vi "Check for Errors.vi"(8 "error in":errorcluster, 11 "Engine in":refnum<class "Engine.lvclass">) -> (0 "error out":errorcluster, 3 "Engine out":refnum<class "Engine.lvclass">)   [LabVIEW 2023, in "Engine.lvlib" / "Engine.lvclass"]
doc: "This routine checks incoming error terminals and relays an error event to the fault handler if there is an error, removing the error from the terminal and allowing the software to continue executing\n\n*This VI will allow the error to pass through if the original error event was not created."
uses:
  Project/Engine.lvclass
  C:/Users/Public/Documents/Development/builds/Engine/Actor Framework.lvlibp/1abvi3w/vi.lib/ActorFramework/Actor/Actor.lvclass
  Project/Engine.lvclass/Engine.ctl
  builds/Engine/Actor Framework.lvlibp/1abvi3w/vi.lib/ActorFramework/Actor/Read Actor Label.vi
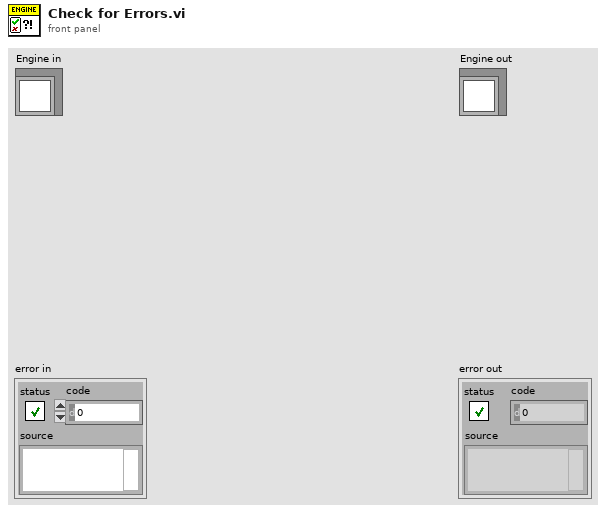
[diagram p1: front panel]
types:
  T1 = cluster{"Accessors:Actor Label":string, "error in ":errorcluster}
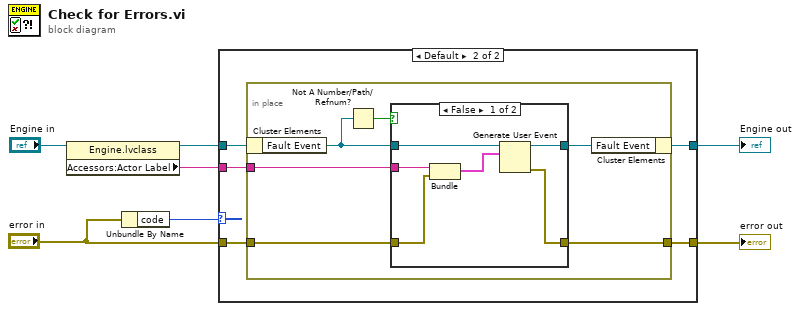
[diagram p0: block diagram]
diagram:
  n1 = property class="Engine.lvclass"(reference="Engine in") -> (reference out=w2:refnum<class "Engine.lvclass">, "Accessors:Actor Label"=w1:string)  [unwired: 1 in, 1 out]
  n2 = Unbundle By Name("error in") -> ("code"=w5:i32)
  n3 = case shown="Default" w5 {
    tunnel: w2 -> [w9 w14]
    tunnel: [w9 w13] -> w6
    tunnel: "error in" -> [w8 w12]
    tunnel: [w8 w11] -> w3
    tunnel: w1 -> [_ w10]
    frame 0 {
    }
    frame Default {
      n4 = in-place {
        in-place-border: w12 -> [w19]
        in-place-border: [w18] -> w11
        in-place-border: w10 -> [w15]
        n5 = in-place-cluster #1(w14) -> ("Fault Event"=w17:refnum<user-event>)
        n6 = Not A Number/Path/Refnum?(number/path/refnum=w17) -> (NaN/Path/Refnum?=w16:bool)
        n7 = case shown="False" w16 {
          tunnel: [w26 w28] -> w20
          tunnel: w19 -> [w22 w27]
          tunnel: [w25 w27] -> w18
          tunnel: w17 -> [w24 w28]
          tunnel: w15 -> [w23 _]
          frame False {
            n8 = Bundle("Accessors:Actor Label"=w23, "error in"=w22) -> (w21:T1)  [unwired: 1 in]
            n9 = Generate User Event(user event=w24, event data cluster=w21) -> (user event out=w26:refnum<user-event>, error out=w25:errorcluster)  [unwired: 2 in]
          }
          frame True {
          }
        }
        n10 = in-place-cluster #1("Fault Event"=w20) -> (w13:refnum<class "Engine.lvclass">)
      }
    }
  }
  "error out" <- w3
  "Engine out" <- w6
